vi "Error Check Empty Ref Array.vi"(8 "error in (no error)":errorcluster, 11 "IDs":u64[](array[numeric])) -> (0 "error out":errorcluster, 3 "IDs dup":u64[](array[numeric]))   [LabVIEW 2020, in "Internal Comm Classes.lvlib" / "WPL Comm.lvclass"]
uses:
  WPL Comm.lvclass
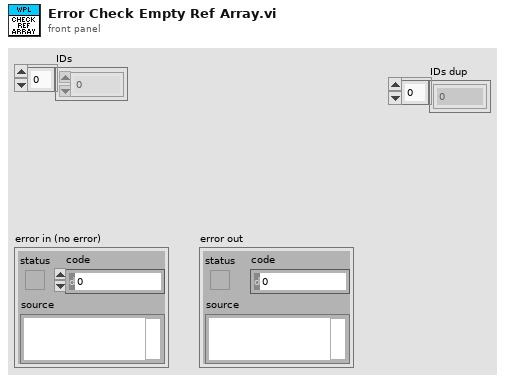
[diagram p1: front panel]
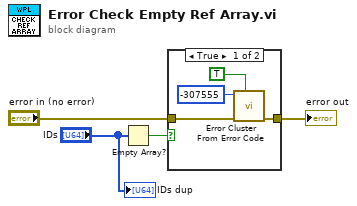
[diagram p0: block diagram]
diagram:
  n1 = Empty Array?(array="IDs") -> (empty?=w1:bool)
  n2 = case shown="True" w1 {
    tunnel: "error in (no error)" -> [w8 w9]
    tunnel: [w6 w9] -> w4
    frame True {
      n3 = call <vilib>:"Error Cluster From Error Code.vi"("show call chain? (False)"=TRUE, "error in (no error)"=w8, "error code (0)"=-307555) -> ("error out"=w6:errorcluster)  [unwired: 6 in]
    }
    frame False {
    }
  }
  "error out" <- w4
  "IDs dup" <- "IDs"
